vi "Enable State.vi"(8 "error in (no error)":errorcluster, 10 "DigNum Refnum":refnum<vi>, 11 "Slide in":refnum<vi>) -> (0 "error out":errorcluster)   [LabVIEW 2018]
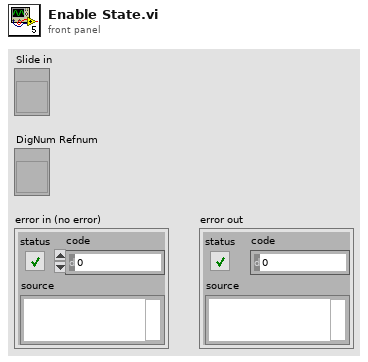
[diagram p1: front panel]
types:
  T1 = enum8{"Enabled", "Disabled", "Disabled and Grayed Out"}
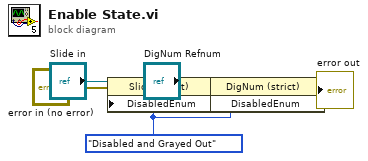
[diagram p0: block diagram]
diagram:
  w6 = T1."Disabled and Grayed Out" ("Disabled")
  n1 = property on="Property Node" class="Slide (strict)"(reference="Slide in", error in="error in (no error)", "DisabledEnum"=w6) -> (error out=w4:errorcluster)  [unwired: 1 out]
  n2 = property on="Property Node" class="DigNum (strict)"(reference="DigNum Refnum", error in=w4, "DisabledEnum"=w6) -> (error out=→"error out":errorcluster)  [unwired: 1 out]
